vi "[C] Log To File.vi"() -> ()   [LabVIEW 2014]
uses:
  <userlib>/_OpenG.lib/file/file.llb/Build Path - Traditional__ogtk.vi
panel:
  in  "Database File":path=path "C:/Users/minister/Documents/GitHub/uf-weather-tower/New Model/database.txt"
  # "INPUT PARAMETERS"
  # "INTERNAL VARIABLES - could possibly be set programatically..."
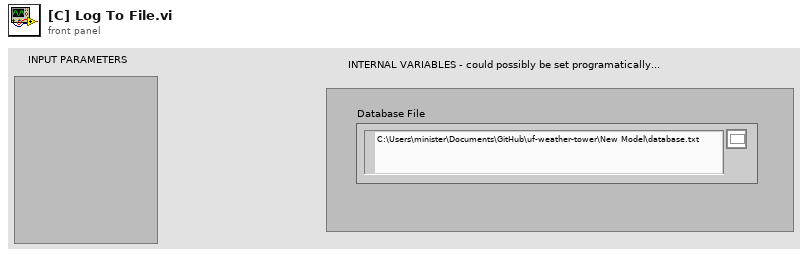
[diagram p1: front panel]
types:
  T1 = enum16{"open", "replace", "create", "open or create", "replace or create", "replace or create with confirmation"}
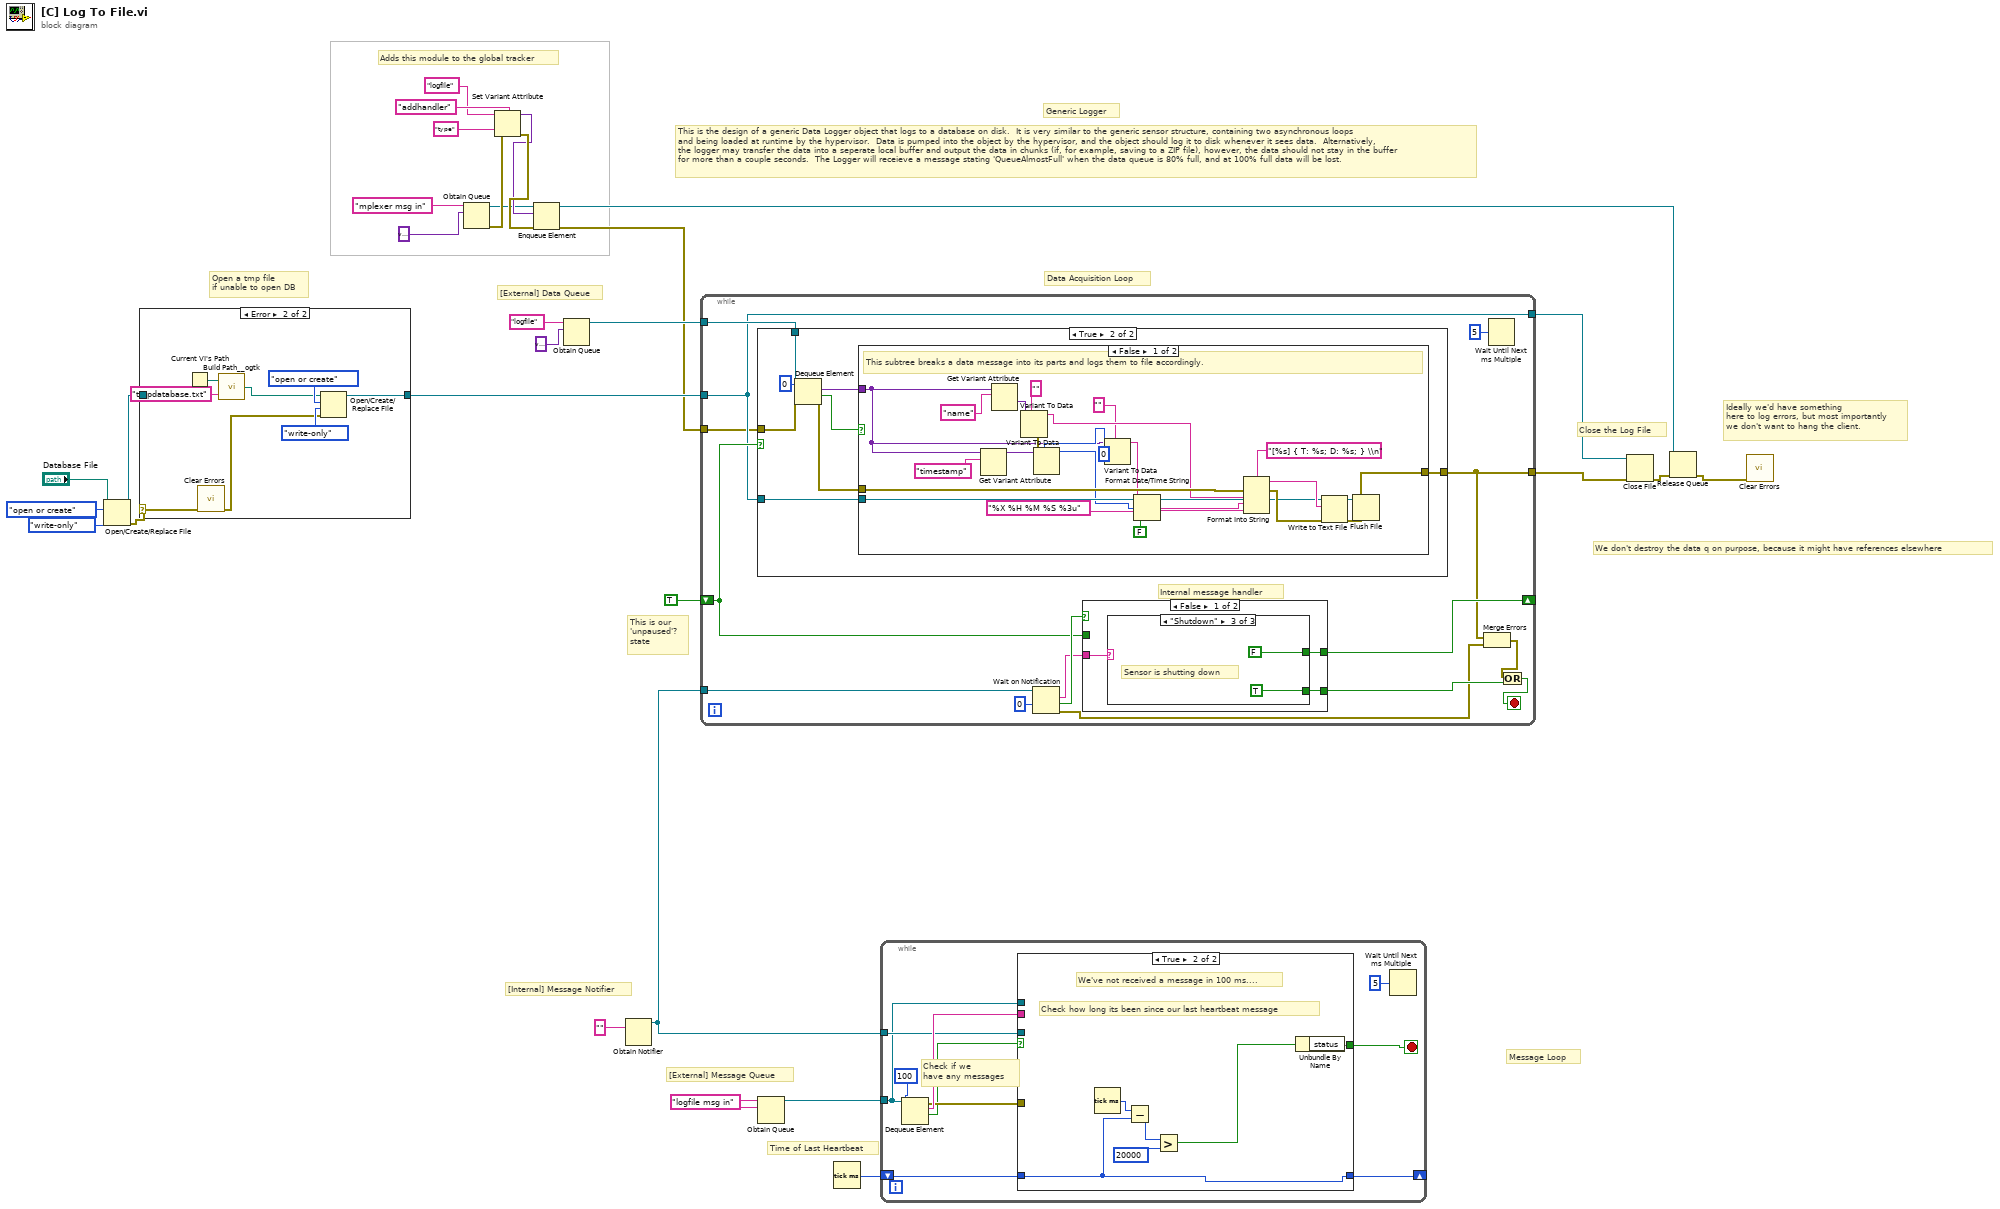
[diagram p0: block diagram]
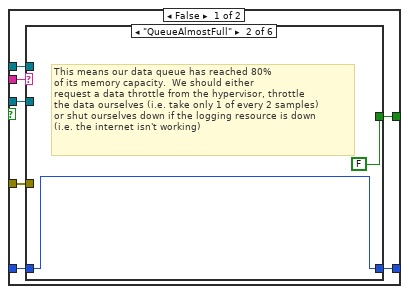
[diagram p3: hidden frame]
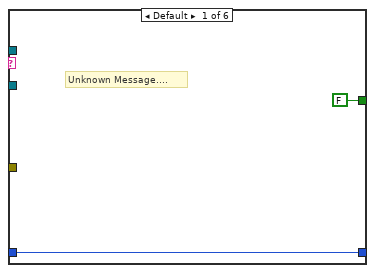
[diagram p4: hidden frame]
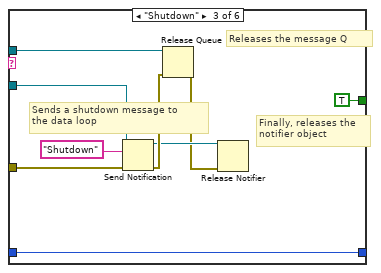
[diagram p5: hidden frame]
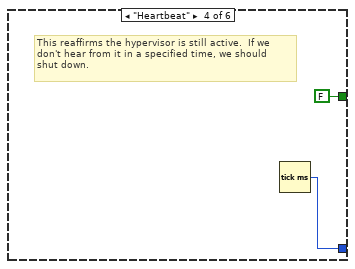
[diagram p6: hidden frame]
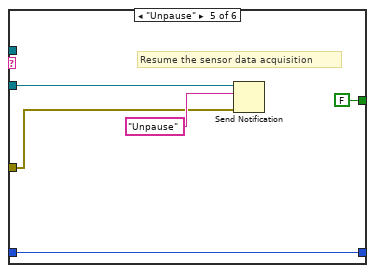
[diagram p7: hidden frame]
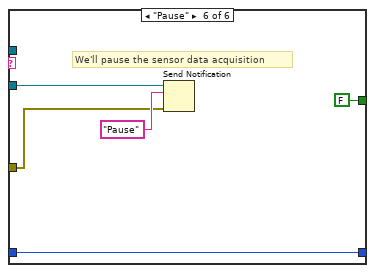
[diagram p8: hidden frame]
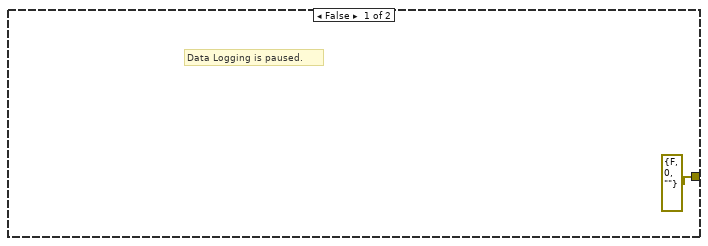
[diagram p9: hidden frame]
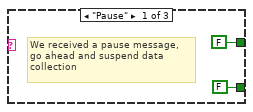
[diagram p11: hidden frame]
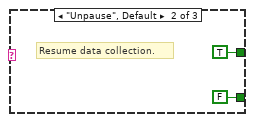
[diagram p12: hidden frame]
diagram:
  w14 = "logfile msg in" ("name (unnamed)")
  # "Message Loop"
  # "Adds this module to the global tracker"
  # "Ideally we'd have something \nhere to log errors, but most importantly\nwe don't want to hang the client."
  # "Time of Last Heartbeat"
  # "Close the Log File"
  # "Open a tmp file\nif unable to open DB"
  # "This is the design of a generic Data Logger object that logs to a database on disk.  It is very similar to the generic sensor structure, containing two asynchronous loops\nand being loaded at runtime by the hypervisor.  Data is pumped into the object by the hypervisor, and the object should log it to disk whenever it sees data.  Alternatively,\nthe logger may transfer the data into a seperate local buffer and output the data in chunks (if, for example, saving to a ZIP file), however, the data should not stay in the buffer\nfor more than a couple seconds.  The Logger will receieve a message stating 'QueueAlmostFull' when the data queue is 80% full, and at 100% full data will be lost."
  # "This is our\n'unpaused'?\nstate"
  # "We don't destroy the data q on purpose, because it might have references elsewhere"
  # "Data Acquisition Loop"
  # "[Internal] Message Notifier"
  # "[External] Message Queue"
  # "[External] Data Queue"
  # "Generic Logger"
  n1 = Open/Create/Replace File(file path (use dialog)="Database File", operation (0:open)=T1."open or create", access (0:read/write)=enum16{"read/write", "read-only", "write-only"}."write-only") -> (refnum out=w23:refnum<file>, error out=w24:errorcluster)  [unwired: 3 in, 1 out]
  n2 = case shown="Error" w24 {
    selector: w24 -> [_ w33]
    tunnel: w23 -> [w31 _]
    tunnel: [w31 w37] -> w22
    frame No Error {
    }
    frame Error {
      n3 = Current VI's Path() -> (path=w36:path)
      n4 = call <vilib>:"Clear Errors.vi"("error in (no error)"=w33) -> ("error out"=w32:errorcluster)  [unwired: 5 in, 1 out]
      n5 = call-poly <userlib>:"Build Path__ogtk.vi"("name or relative path"="tmpdatabase.txt", "base path"=w36) -> ("appended path"=w34:path)
      n6 = Open/Create/Replace File(file path (use dialog)=w34, error in=w32, operation (0:open)=T1."open or create", access (0:read/write)=enum16{"read/write", "read-only", "write-only"}."write-only") -> (refnum out=w37:refnum<file>)  [unwired: 2 in, 2 out]
    }
  }
  n7 = Obtain Queue(name (unnamed)="mplexer msg in", element data type=variant) -> (queue out=w5:refnum<queue>, error out=w8:errorcluster)  [unwired: 3 in, 1 out]
  n8 = Set Variant Attribute(Variant="logfile" ("name"), name="type", value="addhandler" ("name"), error in=w8) -> (Variant out=w6:variant, error out=w7:errorcluster)  [unwired: 1 out]
  n9 = Enqueue Element(queue=w5, element=w6, error in (no error)=w7) -> (queue out=w1:refnum<queue>, error out=w4:errorcluster)  [unwired: 1 in, 1 out]
  n10 = Obtain Queue(name (unnamed)="logfile", element data type=variant) -> (queue out=w16:refnum<queue>)  [unwired: 3 in, 2 out]
  n11 = Obtain Notifier(notification data type="") -> (notifier out=w30:refnum<notifier>)  [unwired: 3 in, 2 out]
  n12 = while {
    tunnel: w16 -> [w45]
    tunnel: w30 -> [w54]
    shift-right: [w50] -> _
    shift-left: TRUE -> [w49]
    tunnel: w22 -> [w44]
    tunnel: [w44] -> w21
    tunnel: [w43] -> w20
    tunnel: w4 -> [w40]
    stop <- w47 stop-if-true
    # "Internal message handler"
    n13 = case shown="True" w49 {
      tunnel: w45 -> [_ w63]
      tunnel: w44 -> [_ w59]
      tunnel: [errorcluster {"status"=FALSE, "code"=0, "source"=""} ("error out") w58] -> w43
      tunnel: w40 -> [_ w56]
      frame False {
        # "Data Logging is paused."
      }
      frame True {
        n14 = Dequeue Element(queue=w63, timeout in ms (-1)=0, error in (no error)=w56) -> (element=w60:variant, timed out?=w61:bool, error out=w57:errorcluster)  [unwired: 1 out]
        n15 = case shown="False" w61 {
          tunnel: w60 -> [w68 _]
          tunnel: w59 -> [w79 _]
          tunnel: [w66 w86] -> w58
          tunnel: w57 -> [w78 w86]
          frame False {
            # "This subtree breaks a data message into its parts and logs them to file accordingly."
            n16 = Get Variant Attribute(Variant=w68, name="timestamp") -> (value=w70:variant)  [unwired: 2 in, 3 out]
            n17 = Get Variant Attribute(Variant=w68, name="name") -> (value=w75:variant)  [unwired: 2 in, 3 out]
            n18 = Variant To Data(type="", Variant=w75) -> (data=w72:string, error out=w74:errorcluster)  [unwired: 1 in]
            n19 = Variant To Data(error in=w74, type=u32 0, Variant=w70) -> (data=w69:u32)  [unwired: 1 out]
            n20 = Variant To Data(type="", Variant=w68) -> (data=w67:string)  [unwired: 1 in, 1 out]
            n21 = Format Date/Time String(time format string (%c)="%X %H %M %S %3u", seconds (now)=w69, UTC format=FALSE) -> (date/time string=w83:string)
            n22 = Format Into String(format string="[%s] { T: %s; D: %s; } \\n", error in=w78, w72, w83, w67) -> (resulting string=w80:string, error out=w81:errorcluster)  [unwired: 1 in]
            n23 = Write to Text File(file (use dialog)=w79, text=w80, error in=w81) -> (refnum out=w65:refnum<file>, error out=w66:errorcluster)  [unwired: 1 in, 1 out]
            n24 = Flush File(refnum=w65, error in=w66) -> ()  [unwired: 2 out]
          }
          frame True {
          }
        }
      }
    }
    n25 = Wait on Notification(notifier=w54, timeout in ms (-1)=0) -> (notification=w51:string, timed out?=w52:bool, error out=w42:errorcluster)  [unwired: 2 in, 1 out]
    n26 = case shown="False" w52 {
      tunnel: w51 -> [w89 _]
      tunnel: [w88 _] -> w48
      tunnel: [w87 w96] -> w50
      tunnel: w49 -> [_ w96]
      frame False {
        n27 = case shown="\"Shutdown\"" w89 {
          tunnel: [FALSE FALSE TRUE] -> w88
          tunnel: [FALSE TRUE FALSE] -> w87
          frame "Pause" {
            # "We received a pause message,\ngo ahead and suspend data collection"
          }
          frame "Unpause", Default {
            # "Resume data collection."
          }
          frame "Shutdown" {
            # "Sensor is shutting down"
          }
        }
      }
      frame True {
      }
    }
    n28 = Merge Errors(w43, w42) -> (w41:errorcluster)
    n29 = Wait Until Next ms Multiple(millisecond multiple=u32 5) -> ()  [unwired: 1 out]
    n30 = Or(x=w41, y=w48) -> (x .or. y?=w47:bool)
  }
  n31 = Obtain Queue(name (unnamed)=w14, element data type=w14) -> (queue out=w15:refnum<queue>)  [unwired: 3 in, 2 out]
  n32 = Tick Count (ms)() -> (millisecond timer value=w19:u32)
  n33 = while {
    tunnel: w15 -> [w103]
    tunnel: w30 -> [w104]
    shift-right: [w98] -> _
    shift-left: w19 -> [w99]
    stop <- w105 stop-if-true
    # "Check if we \nhave any messages"
    n34 = Dequeue Element(queue=w103, timeout in ms (-1)=100) -> (element=w106:string, timed out?=w100:bool, error out=w102:errorcluster)  [unwired: 1 in, 1 out]
    n35 = case shown="True" w100 {
      tunnel: w106 -> [w113 _]
      tunnel: [w112 w140] -> w105
      tunnel: w104 -> [w111 _]
      tunnel: w103 -> [w110 _]
      tunnel: w102 -> [w109 _]
      tunnel: w99 -> [w108 w141]
      tunnel: [w107 w141] -> w98
      frame False {
        n36 = case shown="\"QueueAlmostFull\"" w113 {
          tunnel: [FALSE FALSE TRUE FALSE FALSE FALSE] -> w112
          tunnel: w111 -> [_ _ w124 _ w131 w135]
          tunnel: w110 -> [_ _ w125 _ _ _]
          tunnel: w109 -> [_ _ w123 _ w132 w136]
          tunnel: w108 -> [w114 w116 w118 _ w129 w134]
          tunnel: [w114 w116 w118 w128 w129 w134] -> w107
          frame Default {
            # "Unknown Message...."
          }
          frame "QueueAlmostFull" {
            # "This means our data queue has reached 80%\nof its memory capacity.  We should either\nrequest a data throttle from the hypervisor, throttle\nthe data ourselves (i.e. take only 1 of every 2 samples)\nor shut ourselves down if the logging resource is down\n(i.e. the internet isn't working)"
          }
          frame "Shutdown" {
            # "Finally, releases the\nnotifier object"
            # "Releases the message Q"
            # "Sends a shutdown message to \nthe data loop"
            n37 = Send Notification(notification="Shutdown", notifier=w124, error in (no error)=w123) -> (notifier out=w120:refnum<notifier>, error out=w122:errorcluster)
            n38 = Release Queue(queue=w125, error in (no error)=w122) -> (error out=w119:errorcluster)  [unwired: 1 in, 2 out]
            n39 = Release Notifier(notifier=w120, error in (no error)=w119) -> ()  [unwired: 1 in, 3 out]
          }
          frame "Heartbeat" {
            # "This reaffirms the hypervisor is still active.  If we\ndon't hear from it in a specified time, we should\nshut down."
            n40 = Tick Count (ms)() -> (millisecond timer value=w128:u32)
          }
          frame "Unpause" {
            # "Resume the sensor data acquisition"
            n41 = Send Notification(notification="Unpause", notifier=w131, error in (no error)=w132) -> ()  [unwired: 2 out]
          }
          frame "Pause" {
            # "We'll pause the sensor data acquisition"
            n42 = Send Notification(notification="Pause", notifier=w135, error in (no error)=w136) -> ()  [unwired: 2 out]
          }
        }
      }
      frame True {
        # "Check how long its been since our last heartbeat message"
        # "We've not received a message in 100 ms...."
        n43 = Tick Count (ms)() -> (millisecond timer value=w144:u32)
        n44 = Subtract(x=w144, y=w141) -> (x-y=w143:u32)
        n45 = Greater?(x=w143, y=u32 20000) -> (0:w139:bool)
        n46 = Unbundle By Name(w139) -> ("status"=w140)
      }
    }
    n47 = Wait Until Next ms Multiple(millisecond multiple=u32 5 ("milliseconds to wait")) -> ()  [unwired: 1 out]
  }
  n48 = Close File(refnum=w21, error in=w20) -> (error out=w3:errorcluster)  [unwired: 1 out]
  n49 = Release Queue(queue=w1, error in (no error)=w3) -> (error out=w2:errorcluster)  [unwired: 1 in, 2 out]
  n50 = call <vilib>:"Clear Errors.vi"("error in (no error)"=w2) -> ()  [unwired: 5 in, 2 out]
